vi "Digital Integrator.vi"(0 "Instrument Address":refnum<visa-resource-name>, 1 "Index":i32=-1) -> (2 "dup VISA Session":refnum<visa-resource-name>, 3 "?":dbl[](array[numeric])=[0.00013280642653537187] format="%.4f", 4 "Stop":bool)   [LabVIEW 2019]
doc: "Routine to read the MetroLab PDI 5025 Digital Integrator. Based on routine by Murali Chaparala. Extensively modified, to keep track of rollovers.\nScott Hannahs, NHMFL, December 1994"
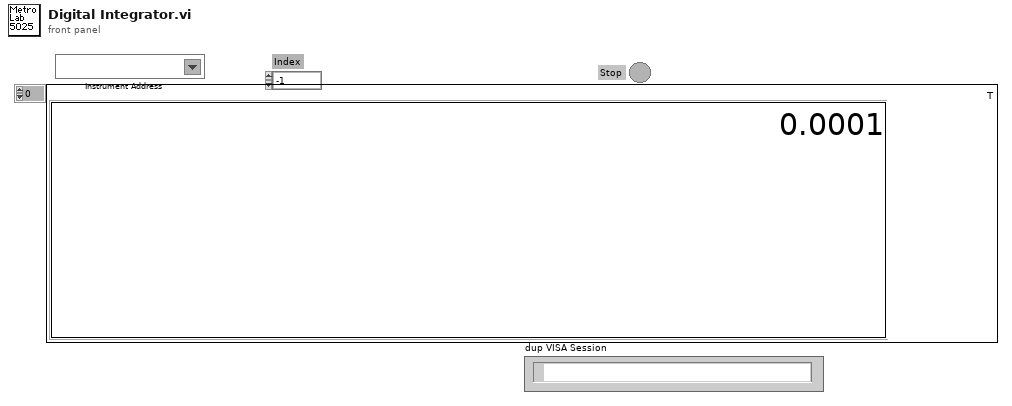
[diagram p1: front panel]
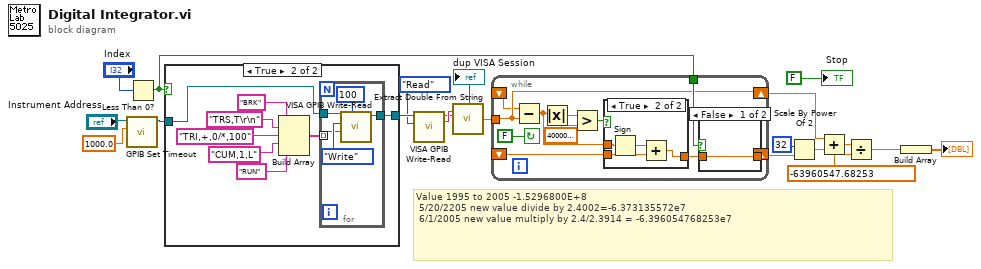
[diagram p0: block diagram]
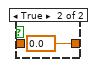
[diagram p2: hidden frame]
diagram:
  # "Value 1995 to 2005 -1.5296800E+8\n 5/20/2205 new value divide by 2.4002=-6.373135572e7\n 6/1/2005 new value multiply by 2.4/2.3914 = -6.396054768253e7"
  n1 = call "GPIB Set Timeout.vi"("Timeout"=sgl 1000.0, "VISA resource name"="Instrument Address") -> ("dup VISA resource name"=w3:refnum<visa-resource-name>)  [unwired: 3 in, 2 out]
  n2 = Less Than 0?(x="Index") -> (x < 0?=w12:bool)
  n3 = case shown="True" w12 {
    tunnel: w3 -> [w20 w21]
    tunnel: [w20 w22] -> w7
    frame False {
    }
    frame True {
      n4 = Build Array("BRK", "TRS,T\r\n", "TRI,+,0/*,100", "CUM,1,L", "RUN") -> (w23:string[])
      n5 = for {
        tunnel: w23 -> [w31] mode=indexing
        tunnel: w21 -> [w33]
        tunnel: [w30] -> w22
        n6 = call "VISA GPIB Write-Read.vi"("Wait (ms)"=u32 100 ("wait (mS)"), "Command"=w31, "Action"=enum16{"Write", "Read", "Write & Read"}."Write", "VISA resource name"=w33) -> ("dup VISA Session"=w30:refnum<visa-resource-name>)  [unwired: 4 in, 3 out]
      }
    }
  }
  n7 = call "VISA GPIB Write-Read.vi"("Action"=enum16{"Write", "Read", "Write & Read"}."Read", "VISA resource name"=w7) -> ("String Returned"=w5:string, "dup VISA Session"=→"dup VISA Session":refnum<visa-resource-name>)  [unwired: 6 in, 2 out]
  n8 = call "Extract Double From String.vi"("string"=w5) -> ("floating pt. number"=w10:dbl)  [unwired: 1 in, 2 out]
  n9 = while {
    tunnel: w10 -> [w36]
    tunnel: w12 -> [w39]
    shift-left: _ -> [w40]
    shift-right: [w37] -> w16
    shift-left: _ -> [w35]
    shift-right: [w36] -> w13
    stop <- FALSE continue-if-true
    n10 = Subtract(x=w35, y=w36) -> (x-y=w41:dbl)
    n11 = Absolute Value(x=w41) -> (abs(x)=w44:dbl)
    n12 = Greater?(x=w44, y=4000000000.0) -> (0:w42:bool)
    n13 = case shown="True" w42 {
      tunnel: w41 -> [_ w51]
      tunnel: w40 -> [w47 w49]
      tunnel: [w47 w48] -> w38
      frame False {
      }
      frame True {
        n14 = Sign(1:w51) -> (0:w50:dbl)
        n15 = Add(x=w50, y=w49) -> (x+y=w48:dbl)
      }
    }
    n16 = case shown="False" w39 {
      tunnel: w38 -> [w45 _]
      tunnel: [w45 0.0] -> w37
      frame False {
      }
      frame True {
      }
    }
  }
  n17 = Scale By Power Of 2(n=32, x=w16) -> (x*2^n=w14:dbl)
  n18 = Add(x=w13, y=w14) -> (x+y=w11:dbl)
  n19 = Divide(x=w11, y=-63960547.68253) -> (x/y=w8:dbl)
  n20 = Build Array(w8) -> (→"?":dbl[])
  "Stop" <- FALSE
